vi "main.vi"() -> ()   [LabVIEW 2024]
uses:
  <vilib>/Instr/_visa.llb/VISA Configure Serial Port (Instr).vi
panel:
  out "俯仰角度":dbl(graph)
  out "方位角度":dbl(graph)
  out "俯仰角度":dbl
  out "方位角度":dbl
  out "COM可用状态":bool
  in  "VISA resource name":refnum<visa-resource-name> caption="COM口选择"
  in  "停止采集":bool
  in  "开始采集":bool
  in  "停止":bool
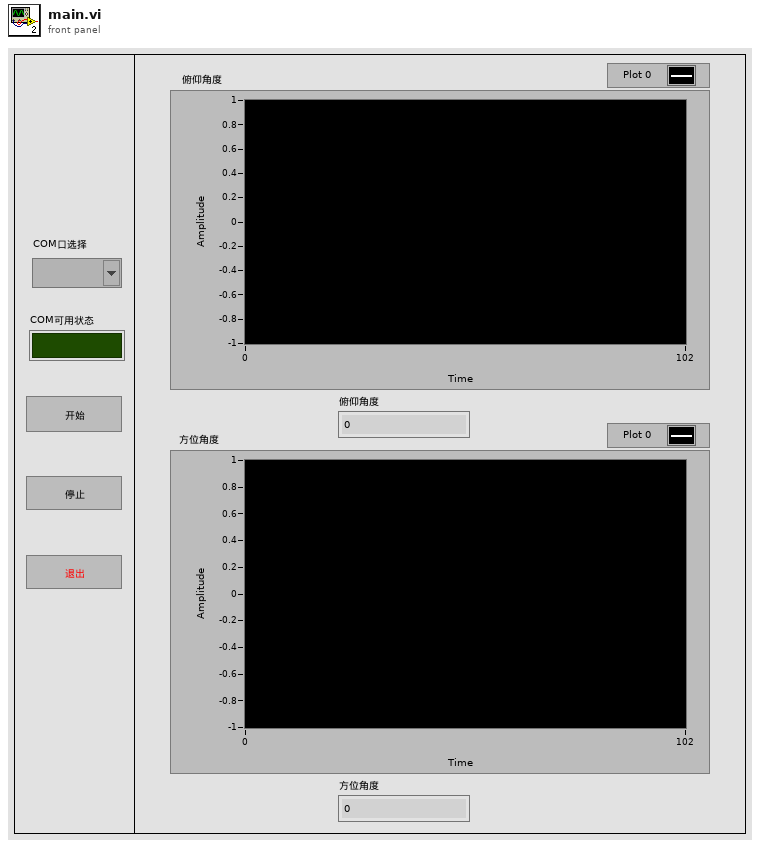
[diagram p1: front panel]
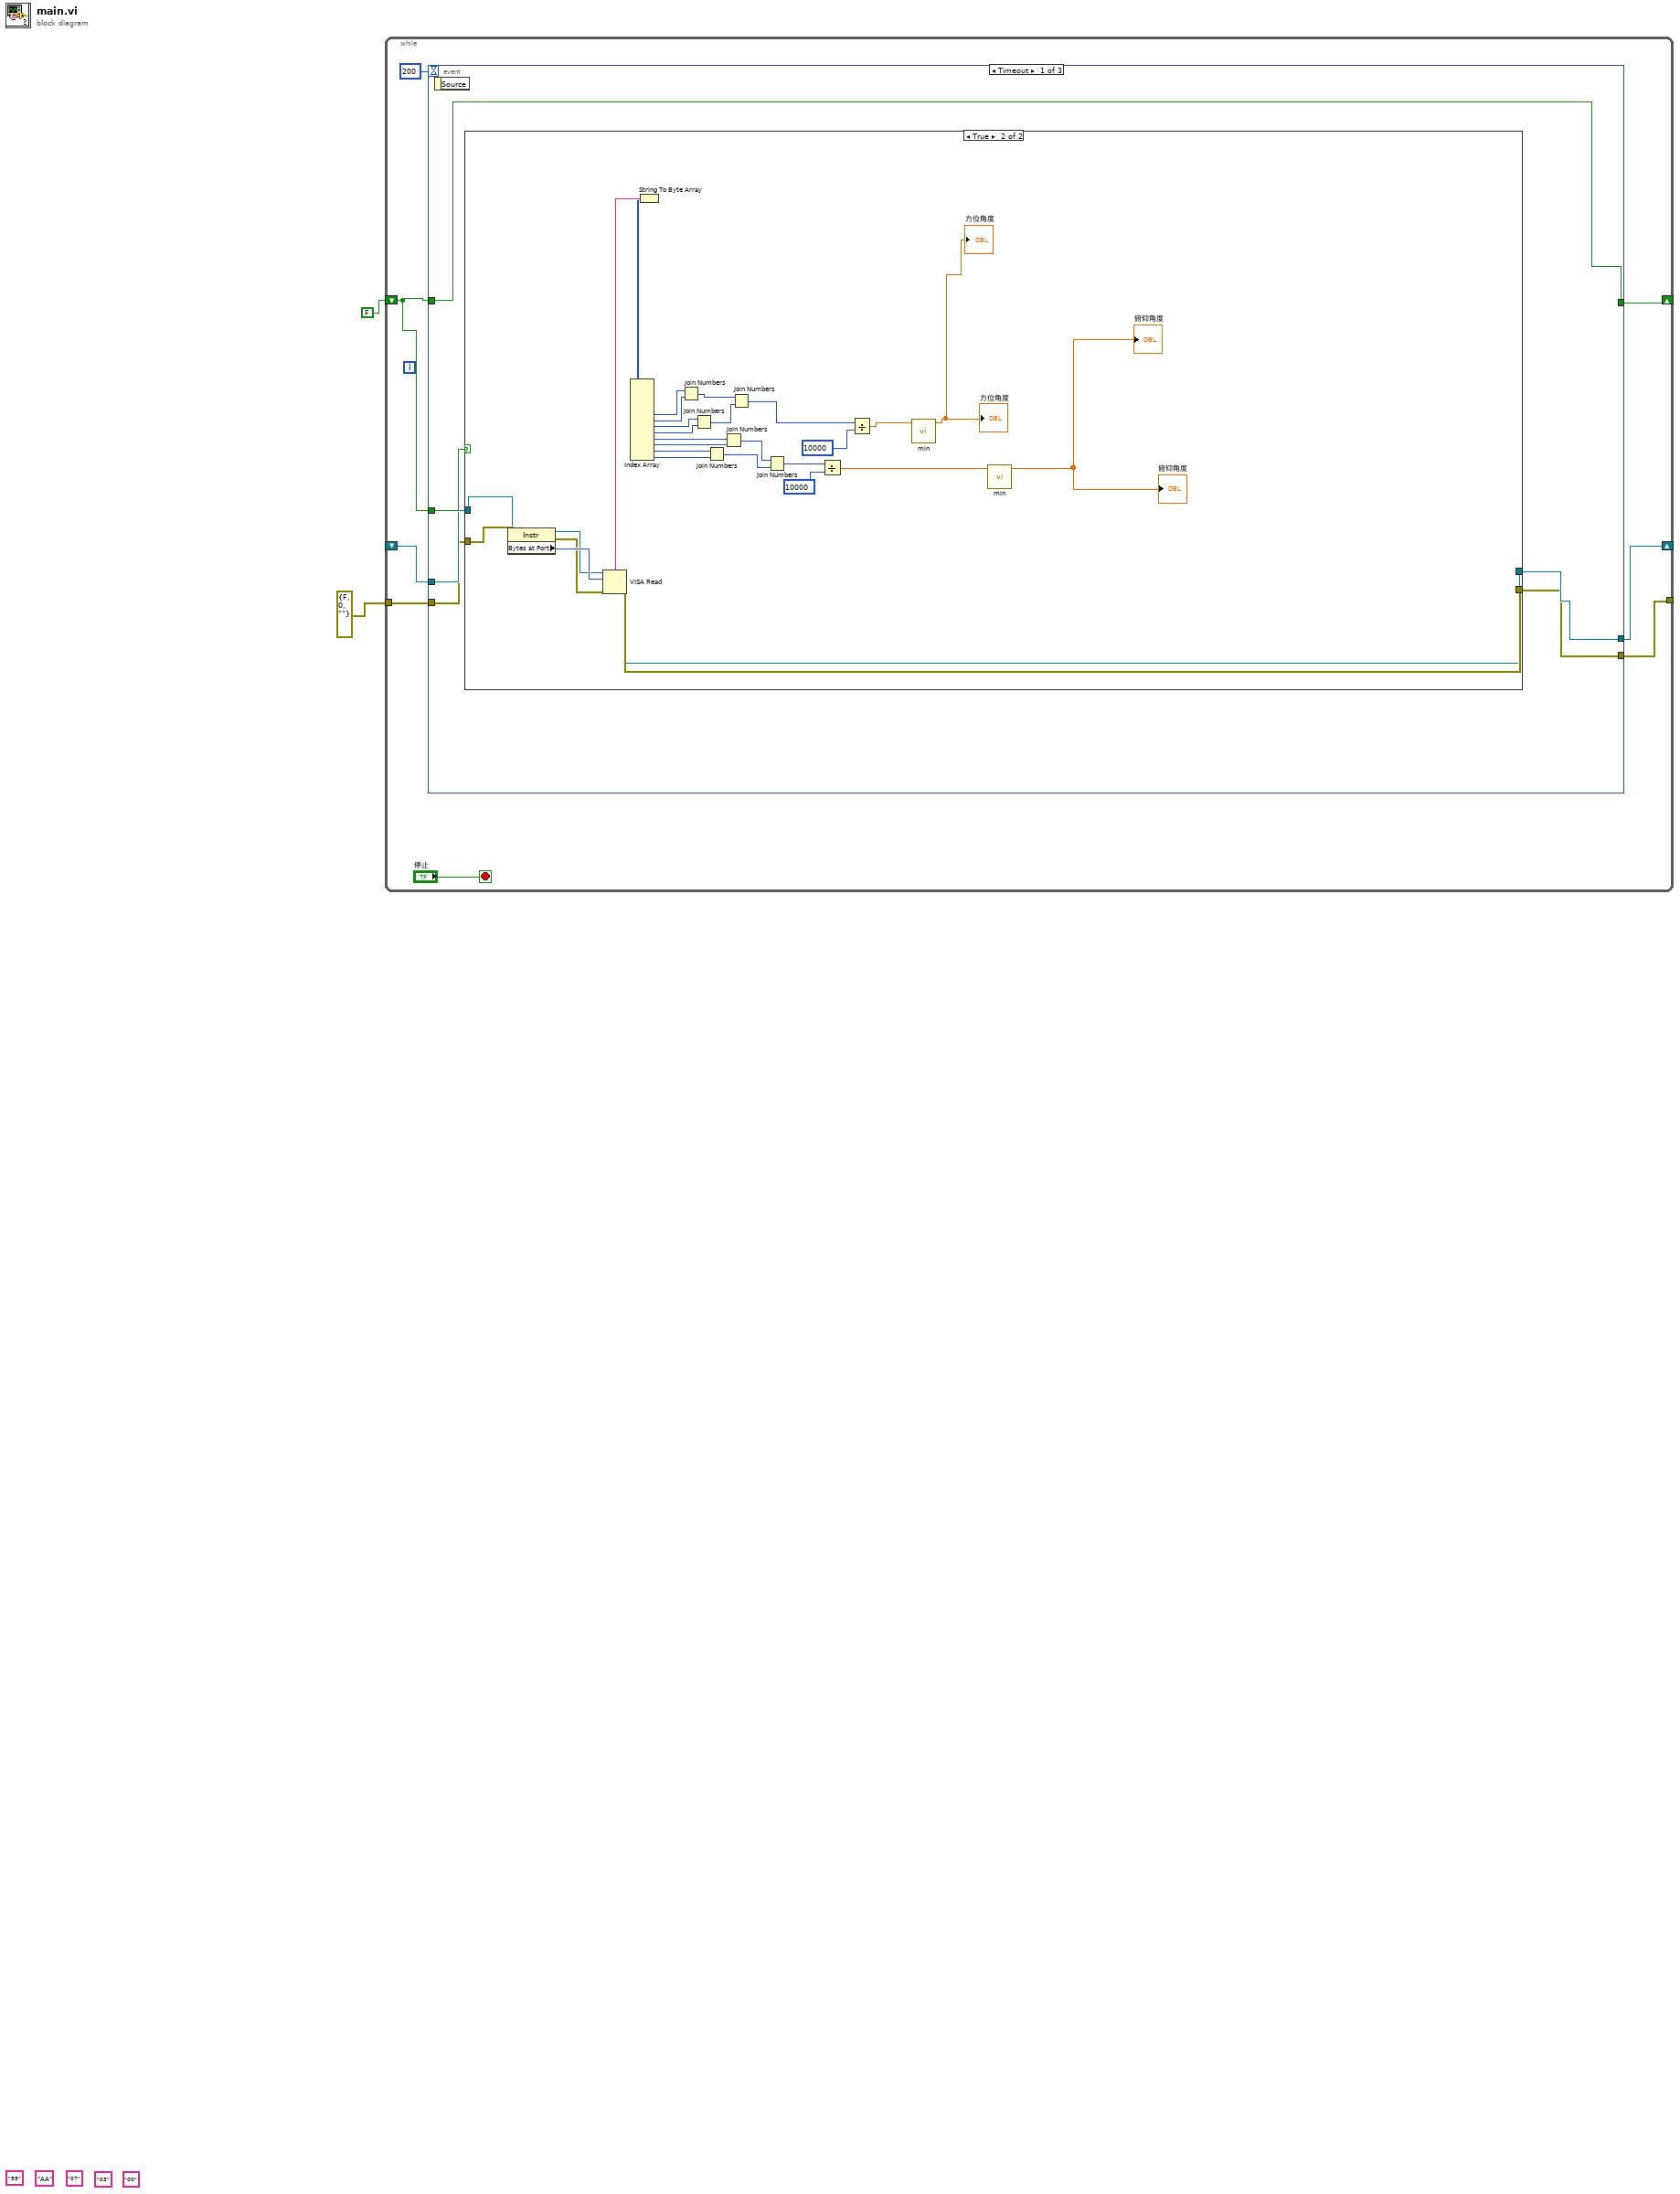
[diagram p0: block diagram]
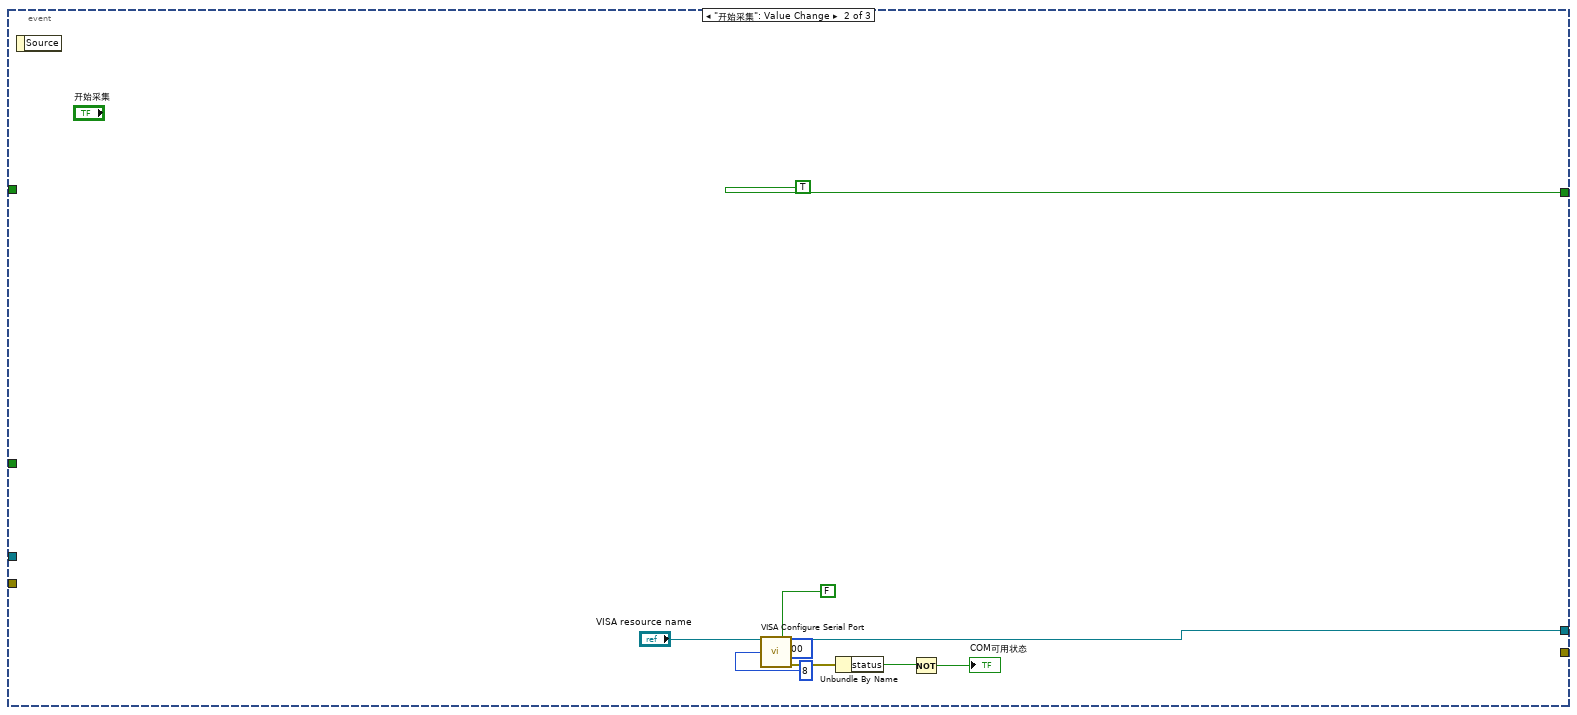
[diagram p3: hidden frame]
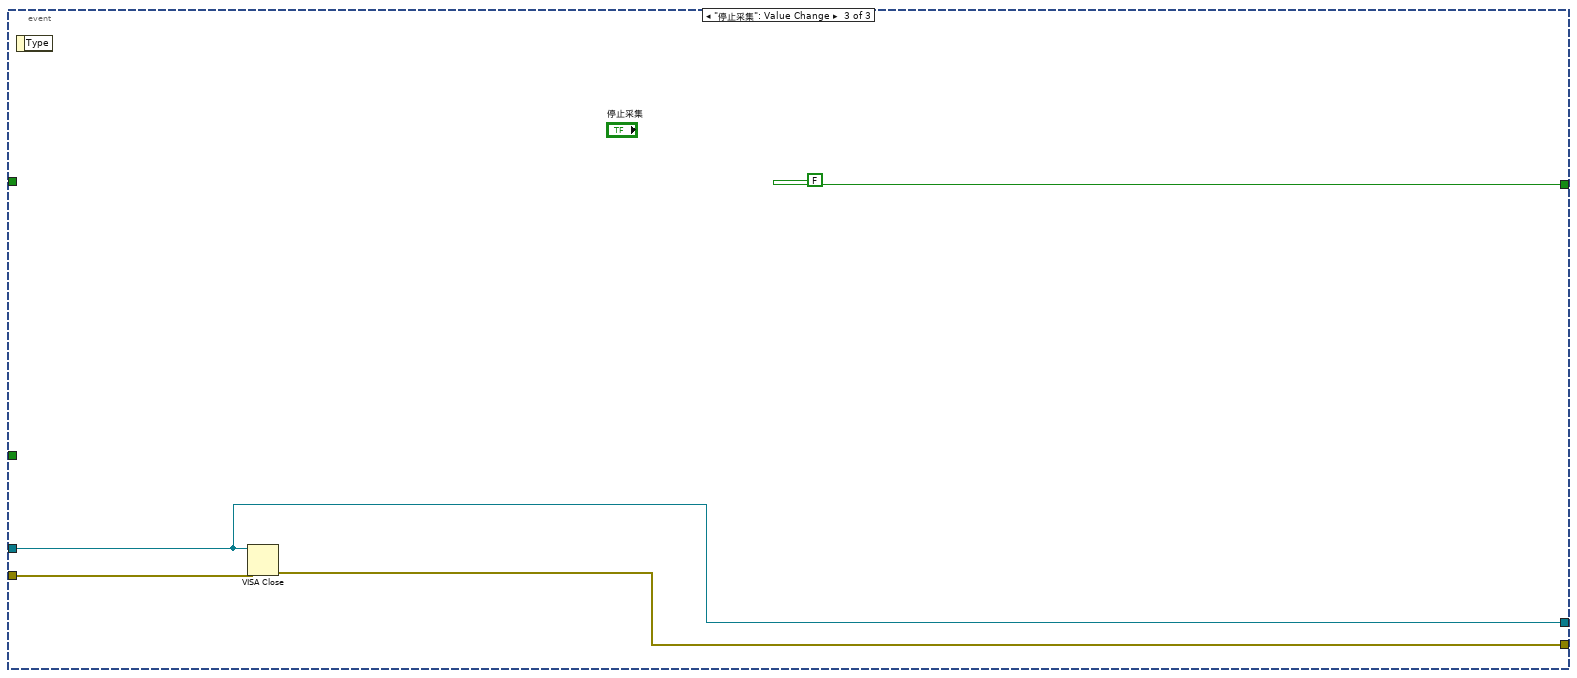
[diagram p4: hidden frame]
diagram:
  (unwired) "00"
  (unwired) "AA"
  (unwired) "07"
  (unwired) "55"
  (unwired) "03"
  n1 = while {
    shift-right: [w8] -> _
    shift-left: FALSE -> [w7]
    shift-right: [w6] -> _
    shift-left: _ -> [w3]
    tunnel: errorcluster {"status"=FALSE, "code"=0, "source"=""} ("错误输入（无错误）") -> [w5]
    tunnel: [w4] -> _
    stop <- "停止" stop-if-true
    n2 = event shown="[0] Timeout" {
      selector: _ -> [_ _ _]
      dyn-events: _ -> [_ _ _]
      timeout: 200 -> [_ _ _]
      tunnel: w7 -> [w16 _ _]
      tunnel: [w15 TRUE ("开始采集") FALSE ("开始采集")] -> w8
      tunnel: w7 -> [w15 _ _]
      tunnel: [w12 w51 w57] -> w6
      tunnel: w3 -> [w14 _ w57]
      tunnel: w5 -> [w13 _ w59]
      tunnel: [w11 _ w58] -> w4
      event Timeout {
        n3 = event-data() -> ()  [unwired: 1 in, 1 out]
        n4 = case shown="True" w16 {
          tunnel: w14 -> [w17 w44]
          tunnel: w13 -> [w18 w47]
          tunnel: [w17 w41] -> w12
          tunnel: [w18 w42] -> w11
          frame False {
          }
          frame True {
            n5 = property class="Instr"(reference=w44, error in=w47) -> (reference out=w43:refnum<visa-resource-name>, error out=w45:errorcluster, "Bytes at Port"=w46:u32)
            n6 = VISA Read(VISA resource name=w43, byte count=w46, error in (no error)=w45) -> (VISA resource name out=w41:refnum<visa-resource-name>, read buffer=w40:string, error out=w42:errorcluster)  [unwired: 1 out]
            n7 = String To Byte Array(string=w40) -> (unsigned byte array=w39:u8[])
            n8 = Index Array(array=w39) -> (element #4=w32:u8, element #5=w31:u8, element #6=w30:u8, element #7=w29:u8, element #8=w25:u8, element #9=w24:u8, element #10=w23:u8, element #11=w22:u8)  [unwired: 11 in, 3 out]
            n9 = Join Numbers(hi=w32, lo=w31) -> ((hi.lo)=w28:u16)
            n10 = Join Numbers(hi=w30, lo=w29) -> ((hi.lo)=w27:u16)
            n11 = Join Numbers(hi=w23, lo=w22) -> ((hi.lo)=w21:u16)
            n12 = Join Numbers(hi=w25, lo=w24) -> ((hi.lo)=w20:u16)
            n13 = Join Numbers(hi=w28, lo=w27) -> ((hi.lo)=w37:u32)
            n14 = Join Numbers(hi=w20, lo=w21) -> ((hi.lo)=w35:u32)
            n15 = Divide(x=w35, y=10000) -> (x/y=w19:dbl)
            n16 = Divide(x=w37, y=10000) -> (x/y=w26:dbl)
            n17 = call "min.vi"("Numeric"=w26) -> ("Numeric 2"=→"方位角度" →"方位角度":dbl)  [unwired: 8 in]
            n18 = call "min.vi"("Numeric"=w19) -> ("Numeric 2"=→"俯仰角度" →"俯仰角度":dbl)  [unwired: 8 in]
          }
        }
      }
      event "开始采集": Value Change {
        n19 = event-data() -> ()  [unwired: 1 in, 1 out]
        n20 = call-poly "VISA Configure Serial Port"("VISA resource name"="VISA resource name", "Enable Termination\nChar (T)"=FALSE, "baud rate (9600)"=u32 460800, "data bits (8)"=u16 8) -> ("VISA resource name out"=w51:refnum<visa-resource-name>, "error out"=w54:errorcluster)  [unwired: 10 in]
        n21 = Unbundle By Name(w54) -> ("status"=w53:bool)
        n22 = Not(x=w53) -> (.not. x?=→"COM可用状态":bool)
      }
      event "停止采集": Value Change {
        n23 = event-data() -> ()  [unwired: 1 in, 1 out]
        n24 = VISA Close(VISA resource name=w57, error in (no error)=w59) -> (error out=w58:errorcluster)
      }
    }
  }
